vi "Set Window Title using Path.vi"(0 "VI path":path, 1 "Title Bar":refnum<vi>, 2 "EXE?":bool, 5 "File Path":path, 9 "Title":string) -> (4 "Title":string)   [LabVIEW 2023]
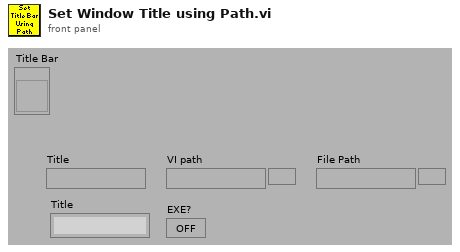
[diagram p1: front panel]
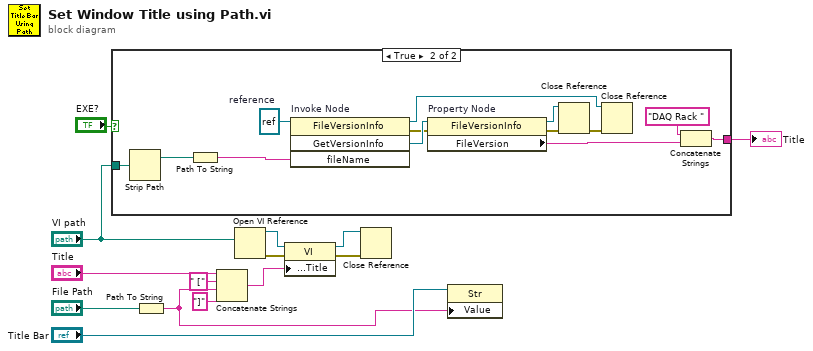
[diagram p0: block diagram]
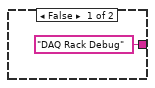
[diagram p2: hidden frame]
diagram:
  n1 = case shown="True" "EXE?" {
    tunnel: "VI path" -> [_ w19]
    tunnel: ["DAQ Rack Debug" w16] -> w5
    frame False {
    }
    frame True {
      w28 = refnum<k24> refnum  # reference
      n2 = Strip Path(path=w19) -> (stripped path=w27:path)  [unwired: 1 out]
      n3 = Path To String(path=w27) -> (string=w26:string)
      n4 = invoke on="Invoke Node" class="FileVersionInfo" method="GetVersionInfo"(reference=w28, "fileName"=w26) -> (reference out=w20:refnum<k24>, error out=w24:errorcluster, "GetVersionInfo"=w25:refnum<k24>)  [unwired: 2 in, 1 out]
      n5 = property on="Property Node" class="FileVersionInfo"(reference=w25, error in=w24) -> (reference out=w23:refnum<k24>, error out=w22:errorcluster, "FileVersion"=w18:string)
      n6 = Close Reference(reference=w23, error in (no error)=w22) -> (error out=w21:errorcluster)
      n7 = Close Reference(reference=w20, error in (no error)=w21) -> ()  [unwired: 1 out]
      n8 = Concatenate Strings("DAQ Rack " ("string"), w18) -> (w16:string)
    }
  }
  "Title" <- w5
  n9 = Path To String(path="File Path") -> (string=w1:string)
  n10 = Concatenate Strings("Title", " [" ("string"), w1, "]" ("string")) -> (w2:string)
  n11 = Open VI Reference(vi path="VI path") -> (vi reference=w11:refnum<vi>, error out=w9:errorcluster)  [unwired: 5 in]
  n12 = property class="VI"(reference=w11, error in=w9, "Front Panel Window:Title"=w2) -> (reference out=w10:refnum<vi>, error out=w8:errorcluster)
  n13 = Close Reference(reference=w10, error in (no error)=w8) -> ()  [unwired: 1 out]
  n14 = property class="Str"(reference="Title Bar", "Value"=w1) -> ()  [unwired: 1 in, 2 out]
